vi "shared-dependency-declareself&takeowner-test.vi"(8 "error in (no error)":errorcluster) -> (0 "error out":errorcluster)   [LabVIEW 2013]
uses:
  _test-support-SMOs/SMO.SelfTerminatingOverride/SMO.SelfTerminatingOverride.lvclass
  _test-support-SMOs/SMO.C/SMO.C.lvclass
  src/SMO/SMO.lvclass
  <vilib>/addons/_JKI Toolkits/Caraya/classes/Assert/Assert.lvclass
  <vilib>/addons/_JKI Toolkits/Caraya/classes/Test/Test.lvclass
  src/Registry/Registry-SMO.lvclass
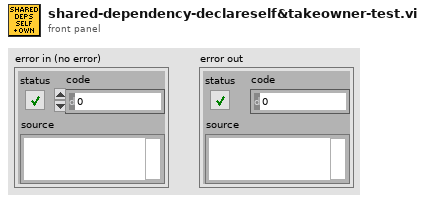
[diagram p1: front panel]
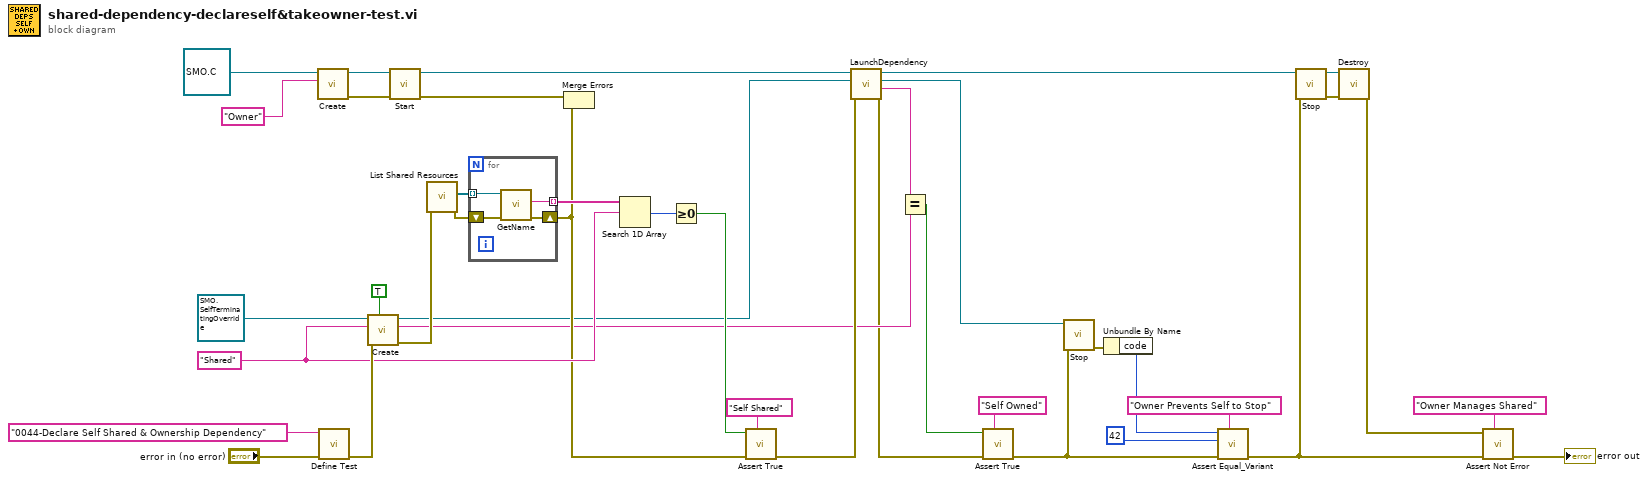
[diagram p0: block diagram]
diagram:
  w25 = "Shared" ("Subsystem Name (optional)")
  n1 = call "Create.vi"("Subsystem Name (optional)"="Owner", "SMO"=refnum<class "SMO.C.lvclass"> refnum ("SMO.C.lvclass")) -> ("error out"=w26:errorcluster, "SMO out"=w29:refnum<class "SMO.C.lvclass">)  [unwired: 7 in, 1 out]
  n2 = call <vilib>:"Define Test.vi"("error in (no error)"="error in (no error)", "Label (VI Title)"="0044-Declare Self Shared & Ownership Dependency") -> ("error out"=w36:errorcluster)  [unwired: 9 in]
  n3 = call "Create.vi"("Shared Resource (F)"=TRUE, "error in (no error)"=w36, "Subsystem Name (optional)"=w25, "SMO"=refnum<class "SMO.SelfTerminatingOverride.lvclass"> refnum ("SMO.SelfTerminatingOverride.lvclass")) -> ("error out"=w23:errorcluster, "SMO name"=w18:string, "SMO out"=w20:refnum<class "SMO.SelfTerminatingOverride.lvclass">)  [unwired: 5 in]
  n4 = call "Start.vi"("error in (no error)"=w26, "SMO"=w29) -> ("error out"=w22:errorcluster, "SMO out"=w24:refnum<class "SMO.C.lvclass">)  [unwired: 8 in]
  n5 = call "List Shared Resources.vi"("error in (no error)"=w23) -> ("error out"=w34:errorcluster, "Shared Resources"=w35:refnum<class "SMO.lvclass">[])  [unwired: 9 in]
  n6 = for {
    tunnel: w35 -> [w44] mode=indexing
    tunnel: [w43] -> w33 mode=indexing
    shift-right: [w41] -> w21
    shift-left: w34 -> [w42]
    n7 = call "GetName.vi"("error in (no error)"=w42, "SMO"=w44) -> ("error out"=w41:errorcluster, "Name"=w43:string)  [unwired: 7 in, 1 out]
  }
  n8 = Merge Errors(w22, w21) -> ()  [unwired: 1 out]
  n9 = Search 1D Array(1D array=w33, element=w25) -> (index of element=w32:i32)  [unwired: 1 in]
  n10 = Greater Or Equal To 0?(x=w32) -> (x >= 0?=w31:bool)
  n11 = call <vilib>:"Assert True.vi"("Label"="Self Shared" ("Filter (regex|name)"), "error in (no error)"=w21, "True?"=w31) -> ("error out"=w19:errorcluster)  [unwired: 8 in]
  n12 = call "LaunchDependency.vi"("error in (no error)"=w19, "Dependency Type"=w20, "SMO in"=w24) -> ("error out"=w14:errorcluster, "Unique Name"=w17:string, "Dependency Reference"=w7:refnum<class "SMO.SelfTerminatingOverride.lvclass">, "SMO out"=w13:refnum<class "SMO.C.lvclass">)  [unwired: 5 in]
  n13 = Equal?(x=w17, y=w18) -> (x = y?=w15:bool)
  n14 = call <vilib>:"Assert True.vi"("Label"="Self Owned" ("Filter (regex|name)"), "error in (no error)"=w14, "True?"=w15) -> ("error out"=w4:errorcluster)  [unwired: 8 in]
  n15 = call "Stop.vi"("error in (no error)"=w4, "SMO"=w7) -> ("error out"=w3:errorcluster)  [unwired: 8 in, 1 out]
  n16 = Unbundle By Name(w3) -> ("code"=w2:i32)
  n17 = call <vilib>:"Assert Equal_Variant.vi"("Label"="Owner Prevents Self to Stop" ("Filter (regex|name)"), "error in (no error)"=w4, "Y"=42 ("code"), "X"=w2) -> ("error out"=w5:errorcluster)  [unwired: 7 in]
  n18 = call "Stop.vi"("error in (no error)"=w5, "SMO"=w13) -> ("error out"=w11:errorcluster, "SMO out"=w12:refnum<class "SMO.C.lvclass">)  [unwired: 8 in]
  n19 = call "Destroy.vi"("error in (no error)"=w11, "SMO"=w12) -> ("error out"=w8:errorcluster)  [unwired: 9 in]
  n20 = call <vilib>:"Assert Not Error.vi"("Label"="Owner Manages Shared" ("Filter (regex|name)"), "error in (no error)"=w5, "Not Error?"=w8) -> ("error out"=→"error out":errorcluster)  [unwired: 8 in]
